vi "Execute.vi"(8 "error in (no error)":errorcluster, 9 "Consumer Queues in":T2, 10 "Trig Process Command in":refnum<class "Configure TRIG Process.lvclass">, 11 "Trig Process Data in":T1) -> (0 "error out":errorcluster, 1 "Consumer Queues out":T2, 2 "Stop?":bool, 3 "Trig Process Data out":T1)   [LabVIEW 2019, in "Trig Process.lvlib" / "Configure TRIG Process.lvclass"]
uses:
  Configure TRIG Process.lvclass
  TS Framework/Consumer Queues.ctl
  UI Process/Generic UI Command/Generic UI Process Command.lvclass
  DAC Process/Generic DAC Command/Generic DAC Process Command.lvclass
  Generic Trig Command/Generic Trig Process Command.lvclass
  Trig Process Data.ctl
  TS Framework/TS Framework.lvlib
  Trig Process.lvlib
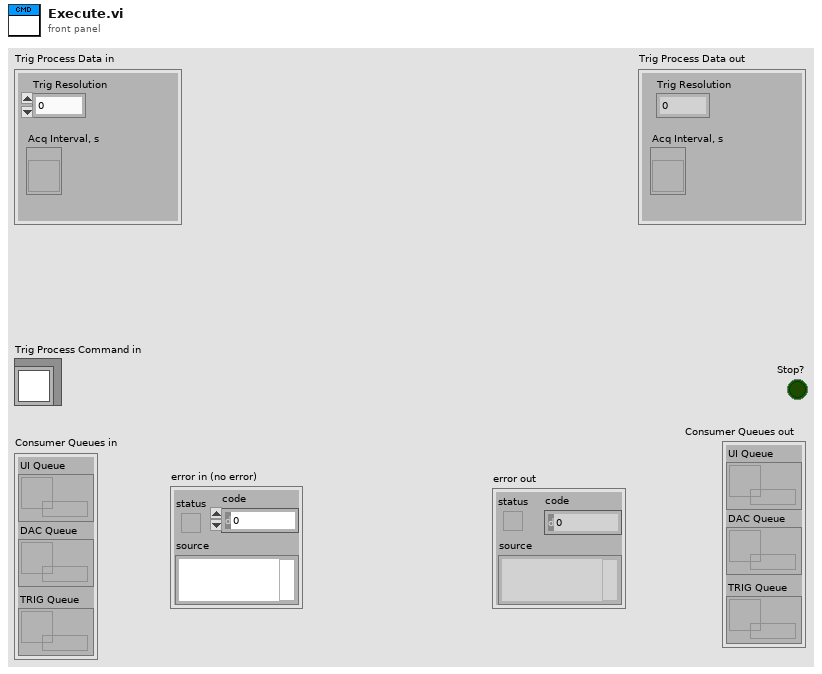
[diagram p1: front panel]
types:
  T1 = typedef "Trig Process.lvlib/Trig Process Data.ctl" = cluster{"Trig Resolution":u32, "Acq Interval":refnum<vi>}
  T2 = typedef "TS Framework.lvlib/Consumer Queues.ctl" = cluster{"UI Queue":refnum<queue>, "DAC Queue":refnum<queue>, "TRIG Queue":refnum<queue>}
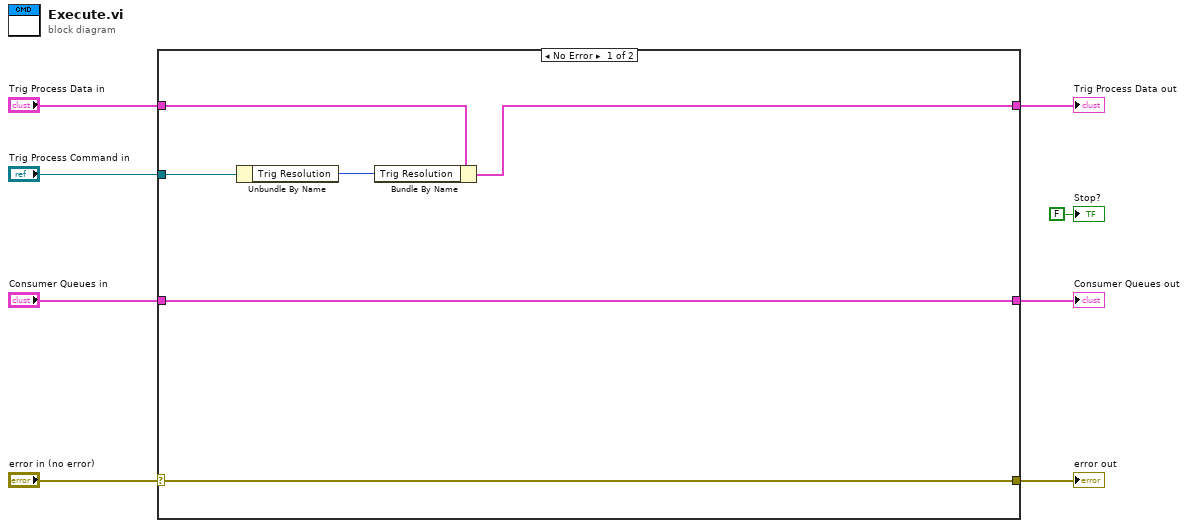
[diagram p0: block diagram]
diagram:
  n1 = case shown="No Error" "error in (no error)" {
    selector: "error in (no error)" -> [w10 w17]
    tunnel: [w10 w17] -> w3
    tunnel: "Consumer Queues in" -> [w9 w16]
    tunnel: [w9 w16] -> w4
    tunnel: "Trig Process Data in" -> [w13 w15]
    tunnel: [w12 w15] -> w5
    tunnel: "Trig Process Command in" -> [w14 _]
    frame No Error {
      n2 = Unbundle By Name(w14) -> ("Trig Resolution"=w11:u32)
      n3 = Bundle By Name(cluster=w13, "Trig Resolution"=w11) -> (w12:T1)
    }
    frame Error {
    }
  }
  "error out" <- w3
  "Consumer Queues out" <- w4
  "Trig Process Data out" <- w5
  "Stop?" <- FALSE ("Stop?")
